vi "Close.vi"(8 "error in":errorcluster, 11 "lia host in":refnum<class "LIA Host Interface RT.lvclass">) -> (0 "error out":errorcluster, 3 "lia host out":refnum<class "LIA Host Interface RT.lvclass">)   [LabVIEW 2018, in "LIA Host Interface RT.lvclass"]
uses:
  LIA Host Interface RT.lvclass
  LIA Host Interface RT.lvclass/LIA Host Interface RT.ctl
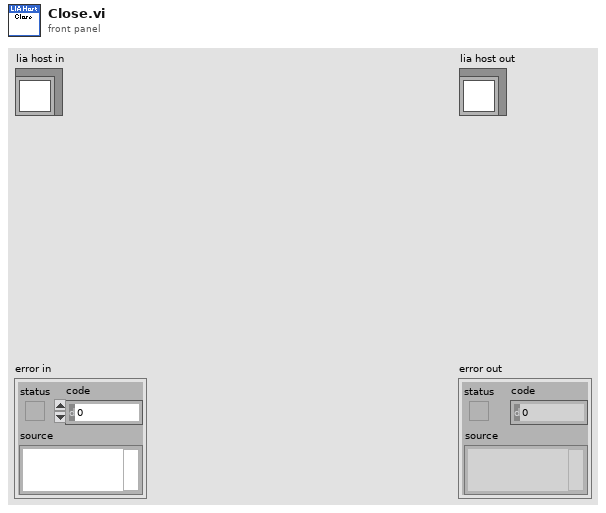
[diagram p1: front panel]
types:
  T1 = typedef "Lock-In Amplifier Host RT.lvclass/session data.ctl" = cluster{"tcp connection":refnum<k5>, "incoming data":refnum<queue>, "outgoing data":refnum<queue>, "lock-in data":refnum<queue>[], "stop process":refnum<notifier>}
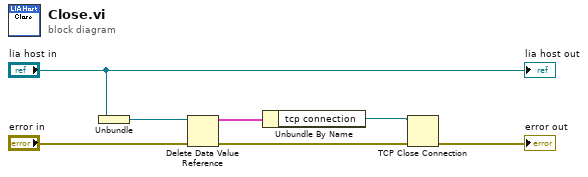
[diagram p0: block diagram]
diagram:
  n1 = Unbundle("lia host in") -> (w6:refnum<data-value>)
  n2 = Delete Data Value Reference(data value reference=w6, error in="error in") -> (data value=w3:T1, error out=w4:errorcluster)
  n3 = Unbundle By Name(w3) -> ("tcp connection"=w1:refnum<k5>)
  n4 = TCP Close Connection(connection ID=w1, error in (no error)=w4) -> (error out=→"error out":errorcluster)  [unwired: 1 in, 1 out]
  "lia host out" <- "lia host in"
